vi "Function Test.vi"(0 "VISA resource name":refnum<visa-resource-name>, 1 "Function Test":u8(ring) items=["OFF", "ON"], 3 "error in":errorcluster, 4 "Enable to Setup":bool, 5 "Enable to Query":bool) -> (7 "VISA resource name out":refnum<visa-resource-name>, 8 "Query the function test status":string, 10 "error out":errorcluster)   [LabVIEW 2011, in "GPT-9000.lvlib"]
uses:
  <instrlib>/GPT-9000/GPT-9000.lvlib
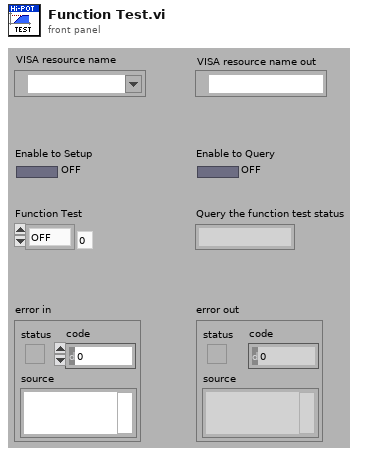
[diagram p1: front panel]
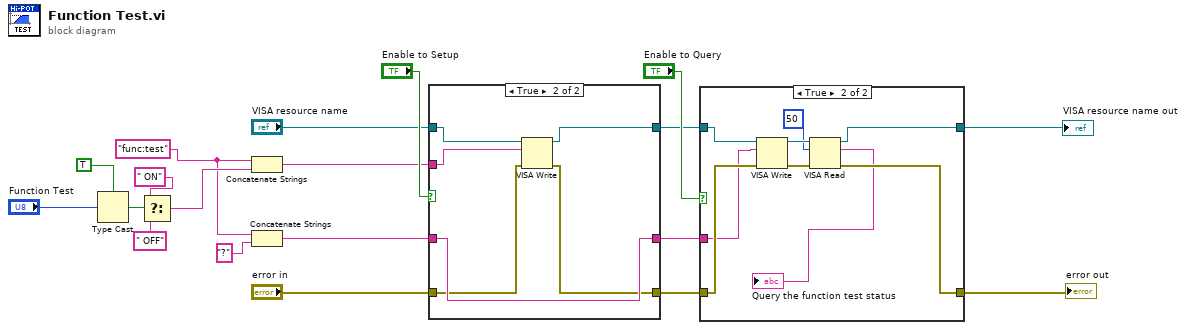
[diagram p0: block diagram]
diagram:
  w10 = "func:test"
  n1 = Type Cast(type=TRUE, x="Function Test") -> (*(type *) &x=w12:bool)
  n2 = Select(t=" ON", s=w12, f=" OFF") -> (s? t:f=w16:string)
  n3 = Concatenate Strings(w10, w16) -> (w8:string)
  n4 = Concatenate Strings(w10, "?" ("string")) -> (w7:string)
  n5 = case shown="True" "Enable to Setup" {
    tunnel: "error in" -> [w21 w25]
    tunnel: "VISA resource name" -> [w22 w27]
    tunnel: [w22 w26] -> w5
    tunnel: [w21 w24] -> w4
    tunnel: w8 -> [_ w23]
    tunnel: w7 -> [w20 w28]
    tunnel: [w20 w28] -> w3
    frame False {
    }
    frame True {
      n6 = VISA Write(VISA resource name=w27, write buffer=w23, error in (no error)=w25) -> (VISA resource name out=w26:refnum<visa-resource-name>, error out=w24:errorcluster)  [unwired: 1 out]
    }
  }
  n7 = case shown="True" "Enable to Query" {
    tunnel: w5 -> [w30 w39]
    tunnel: w4 -> [w29 w38]
    tunnel: w3 -> [_ w37]
    tunnel: [w30 w34] -> w2
    tunnel: [w29 w33] -> w1
    frame False {
    }
    frame True {
      n8 = VISA Write(VISA resource name=w39, write buffer=w37, error in (no error)=w38) -> (VISA resource name out=w36:refnum<visa-resource-name>, error out=w35:errorcluster)  [unwired: 1 out]
      n9 = VISA Read(VISA resource name=w36, byte count=u32 50, error in (no error)=w35) -> (VISA resource name out=w34:refnum<visa-resource-name>, read buffer=→"Query the function test status":string, error out=w33:errorcluster)  [unwired: 1 out]
    }
  }
  "VISA resource name out" <- w2
  "error out" <- w1
